vi "给表格行上色.vi"(6 "列数":i32, 8 "错误输入（无错误）":errorcluster, 9 "颜色":u32(colorbox)=16763272, 10 "行输入":i32, 11 "引用输入":refnum<vi>) -> (0 "错误输出":errorcluster, 2 "行输出":i32, 3 "引用输出":refnum<vi>)   [LabVIEW 2014, in "表格.lvlib"]
uses:
  <vilib>/Utility/miscctls.llb/LVRowAndColumnTypeDef.ctl
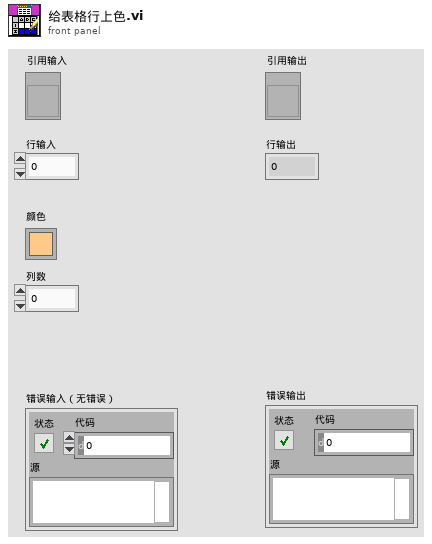
[diagram p1: front panel]
types:
  T1 = typedef "LVRowAndColumnTypeDef.ctl" = cluster{"Row":i32, "Column":i32}
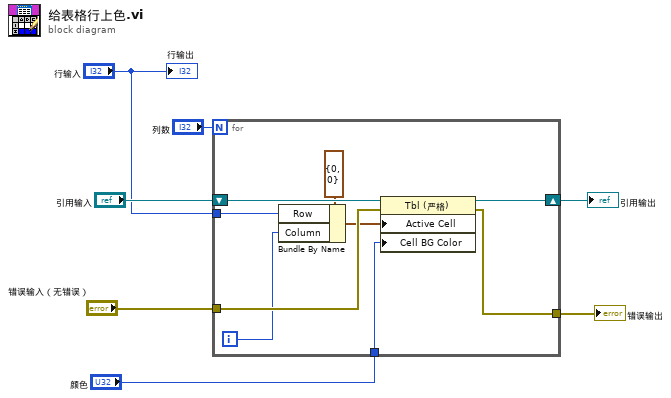
[diagram p0: block diagram]
diagram:
  n1 = for {
    N: "列数" -> [_]
    tunnel: "颜色" -> [w15]
    shift-right: [w14] -> w5
    shift-left: "引用输入" -> [w16]
    tunnel: [w13] -> w4
    tunnel: "错误输入（无错误）" -> [w12]
    tunnel: "行输入" -> [w8]
    i -> [w9]
    n2 = Bundle By Name(cluster=T1 {"Row"=0, "Column"=0} ("上次坐标"), "Row"=w8, "Column"=w9) -> (w10:T1)
    n3 = property on="属性节点" class="Tbl (严格)"(reference=w16, error in=w12, "Active Cell"=w10, "Cell BG Color"=w15) -> (reference out=w14:refnum<vi>, error out=w13:errorcluster)
  }
  "错误输出" <- w4
  "引用输出" <- w5
  "行输出" <- "行输入"
